vi "Aquisicao_Temperatura_e_Velocidade.vi"() -> ()   [LabVIEW 2018]
uses:
  <vilib>/Analysis/8numeric.llb/1D Numeric Integration.vi
  <vilib>/Waveform/WDTOps.llb/WDT Append Waveforms DBL.vi
  <vilib>/Waveform/WDTOps.llb/WDT Number of Waveform Samples DBL.vi
  <vilib>/Analysis/NI_AALPro.lvlib
panel:
  out "Gráfico de aceleração":waveform(dbl)(graph) caption="Gráfico de temperatura"
  out "Temperatura":dbl format="%#.1g"
  out "stop 2":bool
  in  "Velocidade inicial (m/s)":dbl=1.0 caption="Time Target (s)"
  out "Gráfico de velocidade":waveform(dbl)(graph)
  out "Tempo de aquisição máximo (s) 2":dbl caption="Elapsed Time (s)"
  out "Tempo de aquisição 2 (s)":dbl caption="Elapsed Time (s)"
  in  "Frequência de amostragem (Hz)":dbl=1.0 caption="Time Target (s)"
  out "Tempo de aquisição (s)":dbl caption="Elapsed Time (s)"
  in  "OK Button":bool
  in  "stop":bool
  out "Gráfico de temperatura":waveform(dbl)(graph)
  in  "Unidade de temperatura":enum16{"Celsius", "Kelvin"}(ring)
  in  "Tempo de aquisição máximo (s)":dbl=1.0 caption="Time Target (s)"
  # "CÓDIGO PARA AQUISIÇÃO SINCRONIZADA DE TEMPERATURA E VELOCIDADE"
  # "TEMPERATURA"
  # "VELOCIDADE E ACELERA敲O"
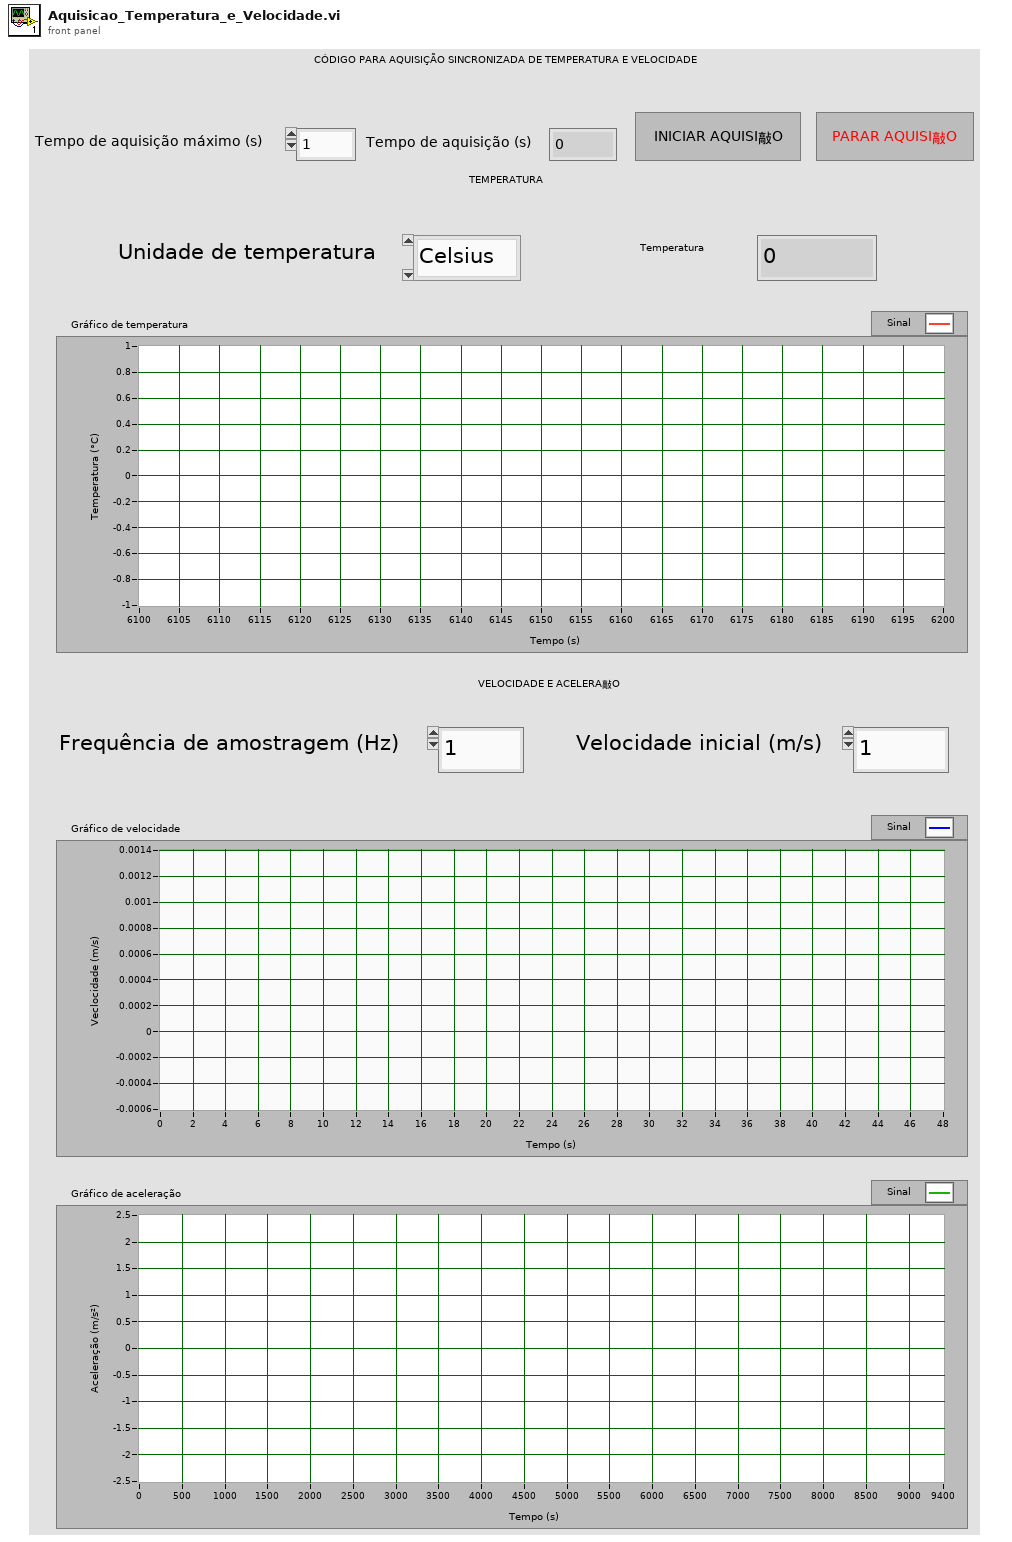
[diagram p1: front panel]
types:
  T1 = typedef "NI_Matrix.lvlib/RealMatrix.ctl" = dbl[][]
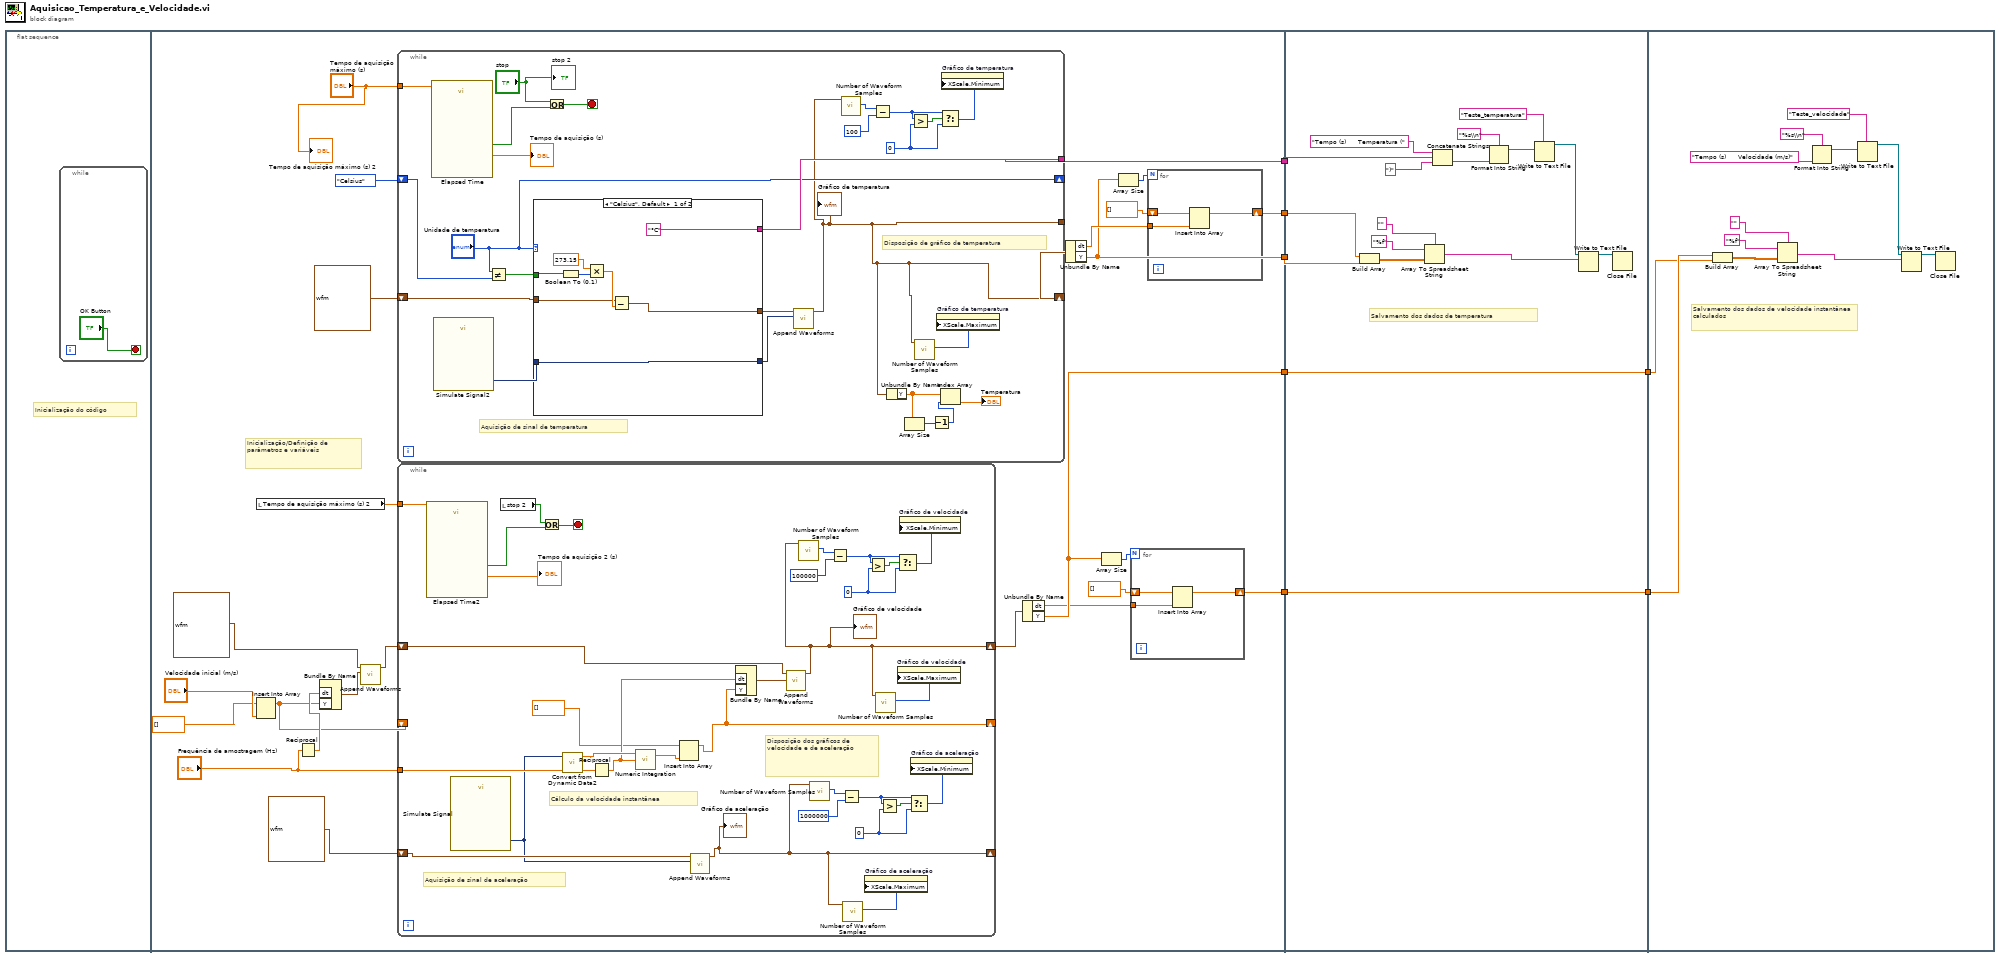
[diagram p0: block diagram]
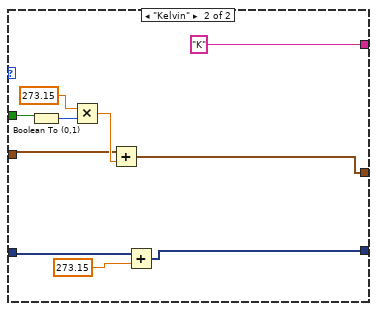
[diagram p2: hidden frame]
diagram:
  n1 = flat-sequence {
    tunnel: [w19] -> w7
    tunnel: [w29] -> w6
    tunnel: [w9] -> w5
    tunnel: [w11] -> w4
    tunnel: [w10] -> w3
    tunnel: w7 -> [w116]
    tunnel: w6 -> [w124]
    tunnel: w5 -> [w118]
    tunnel: w4 -> [w117]
    tunnel: w3 -> [w115]
    tunnel: [w116] -> w2
    tunnel: [w115] -> w1
    tunnel: w2 -> [w132]
    tunnel: w1 -> [w133]
    frame #0 {
      # "Inicialização do código"
      n2 = while {
        stop <- "OK Button" stop-if-true
      }
    }
    frame #1 {
      # "Inicialização/Definição de parâmetros e variáveis"
      n3 = Insert Into Array(array=dbl[] [] ("Y"), new element="Velocidade inicial (m/s)") -> (w23:dbl[])  [unwired: 1 in]
      n4 = local read "Tempo de aquisição máximo (s) 2"() -> (w31:dbl)
      n5 = Reciprocal(x="Frequência de amostragem (Hz)") -> (1/x=w24:dbl)
      n6 = Bundle By Name("dt"=w24, "Y"=w23) -> (w22:waveform(dbl))  [unwired: 1 in]
      n7 = call-poly <vilib>:"Append Waveforms.vi"("waveform B"=w22, "waveform A"=waveform(dbl) {"t0"=timestamp(0 s since 1904-01-01), "dt"=1.0, "Y"=[]}) -> ("waveform out"=w20:waveform(dbl))  [unwired: 8 in, 1 out]
      n8 = while {
        shift-right: [w72] -> w15
        shift-left: waveform(dbl) {"t0"=timestamp(0 s since 1904-01-01), "dt"=1.0, "Y"=[]} ("waveform A") -> [w89]
        tunnel: "Tempo de aquisição máximo (s)" -> [w95]
        shift-right: ["Unidade de temperatura"] -> _
        shift-left: enum16{"Celsius", "Kelvin"}."Celsius" ("Enum") -> [w87]
        tunnel: [w72] -> _
        tunnel: [w93] -> w29
        stop <- w92 stop-if-true
        w75 = 0 ("f")
        # "Disposição de gráfico de temperatura"
        # "Aquisição de sinal de temperatura"
        n9 = call "Elapsed Time"("Time Target (s)"=w95) -> ("Elapsed Time (s)"=→"Tempo de aquisição (s)":dbl, "Time has Elapsed"=w91:bool)  [unwired: 11 in, 6 out]
        n10 = call "Simulate Signal2"() -> ("Sine"=w84:dynamicdata)  [unwired: 14 in, 1 out]
        n11 = Not Equal?(x="Unidade de temperatura", y=w87) -> (x != y?=w86:bool)
        n12 = case shown="\"Celsius\", Default" "Unidade de temperatura" {
          tunnel: ["°C" "K"] -> w93
          tunnel: w89 -> [w99 w105]
          tunnel: [w98 w110] -> w96
          tunnel: w84 -> [w103 w113]
          tunnel: [w103 w112] -> w94
          tunnel: w86 -> [w97 w107]
          frame "Celsius", Default {
            n13 = Boolean To (0,1)(Boolean=w97) -> (0, 1=w101:i16)
            n14 = Multiply(x=273.15 ("y"), y=w101) -> (x*y=w100:dbl)
            n15 = Subtract(x=w99, y=w100) -> (x-y=w98:waveform(dbl))
          }
          frame "Kelvin" {
            n16 = Boolean To (0,1)(Boolean=w107) -> (0, 1=w108:i16)
            n17 = Multiply(x=273.15 ("y"), y=w108) -> (x*y=w106:dbl)
            n18 = Add(x=w105, y=w106) -> (x+y=w110:waveform(dbl))
            n19 = Add(x=w113, y=273.15) -> (x+y=w112:dynamicdata)
          }
        }
        n20 = Or(x="stop", y=w91) -> (x .or. y?=w92:bool)
        n21 = call-poly <vilib>:"Append Waveforms.vi"("waveform B"=w94, "waveform A"=w96) -> ("waveform out"=w72:waveform(dbl))  [unwired: 8 in, 1 out]
        "Gráfico de temperatura" <- w72
        n22 = call-poly <vilib>:"Number of Waveform Samples.vi"("waveform in"=w72) -> ("number of samples"=w79:i32)  [unwired: 8 in, 2 out]
        n23 = Subtract(x=w79, y=100) -> (x-y=w76:i32)
        n24 = Unbundle By Name(w72) -> ("Y"=w83:dbl[])
        n25 = Array Size(array=w83) -> (size(s)=w81:i32)
        n26 = Greater?(x=w76, y=w75) -> (0:w77:bool)
        n27 = call-poly <vilib>:"Number of Waveform Samples.vi"("waveform in"=w72) -> ("number of samples"=w73:i32)  [unwired: 8 in, 2 out]
        n28 = Decrement(x=w81) -> (x-1=w80:i32)
        n29 = property on="Gráfico de temperatura" class="WFGraph (strict)"("XScale.Maximum"=w73) -> ()  [unwired: 2 in, 2 out]
        n30 = Select(t=w76, s=w77, f=w75) -> (s? t:f=w74:i32)
        n31 = Index Array(array=w83, index=w80) -> (element=→"Temperatura":dbl)
        n32 = property on="Gráfico de temperatura" class="WFGraph (strict)"("XScale.Minimum"=w74) -> ()  [unwired: 2 in, 2 out]
        "stop 2" <- "stop"
      }
      n33 = while {
        tunnel: w31 -> [w70]
        tunnel: "Frequência de amostragem (Hz)" -> [w42]
        shift-right: [w51] -> w30
        shift-left: w20 -> [w52]
        shift-right: [w43] -> _
        shift-left: waveform(dbl) {"t0"=timestamp(0 s since 1904-01-01), "dt"=1.0, "Y"=[]} ("waveform A") -> [w66]
        shift-right: [w54] -> _
        shift-left: w23 -> [_]
        stop <- w69 stop-if-true
        w46 = 0 ("f")
        w61 = 0 ("f")
        # "Disposição dos gráficos de velocidade e de aceleração"
        # "Cálculo da velocidade instantânea"
        # "Aquisição de sinal de aceleração"
        n34 = call "Elapsed Time2"("Time Target (s)"=w70) -> ("Elapsed Time (s)"=→"Tempo de aquisição 2 (s)":dbl, "Time has Elapsed"=w71:bool)  [unwired: 11 in, 6 out]
        n35 = call "Simulate Signal"() -> ("Sine with Uniform Noise"=w41:dynamicdata)  [unwired: 14 in, 1 out]
        n36 = local read "stop 2"() -> (w67:bool)
        n37 = Or(x=w67, y=w71) -> (x .or. y?=w69:bool)
        n38 = call "Convert from Dynamic Data2"("Dynamic Data Type"=w41) -> ("Array"=w58:dbl[])  [unwired: 3 in]
        n39 = Reciprocal(x=w42) -> (1/x=w57:dbl)
        n40 = call-poly <vilib>:"Numeric Integration.vi"("dt"=w57, "Input Array"=w58) -> ("result"=w56:dbl)  [unwired: 1 in, 1 out]
        n41 = Insert Into Array(array=dbl[] [] ("Y"), new element=w56) -> (w54:dbl[])  [unwired: 1 in]
        n42 = call-poly <vilib>:"Append Waveforms.vi"("waveform B"=w41, "waveform A"=w66) -> ("waveform out"=w43:waveform(dbl))  [unwired: 8 in, 1 out]
        "Gráfico de aceleração" <- w43
        n43 = Bundle By Name("dt"=w57, "Y"=w54) -> (w53:waveform(dbl))  [unwired: 1 in]
        n44 = call-poly <vilib>:"Append Waveforms.vi"("waveform B"=w53, "waveform A"=w52) -> ("waveform out"=w51:waveform(dbl))  [unwired: 8 in, 1 out]
        "Gráfico de velocidade" <- w51
        n45 = call-poly <vilib>:"Number of Waveform Samples.vi"("waveform in"=w51) -> ("number of samples"=w65:i32)  [unwired: 8 in, 2 out]
        n46 = call-poly <vilib>:"Number of Waveform Samples.vi"("waveform in"=w43) -> ("number of samples"=w50:i32)  [unwired: 8 in, 2 out]
        n47 = Subtract(x=w65, y=100000) -> (x-y=w62:i32)
        n48 = Subtract(x=w50, y=1000000) -> (x-y=w47:i32)
        n49 = call-poly <vilib>:"Number of Waveform Samples.vi"("waveform in"=w43) -> ("number of samples"=w44:i32)  [unwired: 8 in, 2 out]
        n50 = property on="Gráfico de aceleração" class="WFGraph (strict)"("XScale.Maximum"=w44) -> ()  [unwired: 2 in, 2 out]
        n51 = Greater?(x=w62, y=w61) -> (0:w63:bool)
        n52 = call-poly <vilib>:"Number of Waveform Samples.vi"("waveform in"=w51) -> ("number of samples"=w59:i32)  [unwired: 8 in, 2 out]
        n53 = Greater?(x=w47, y=w46) -> (0:w48:bool)
        n54 = property on="Gráfico de velocidade" class="WFGraph (strict)"("XScale.Maximum"=w59) -> ()  [unwired: 2 in, 2 out]
        n55 = Select(t=w62, s=w63, f=w61) -> (s? t:f=w60:i32)
        n56 = property on="Gráfico de velocidade" class="WFGraph (strict)"("XScale.Minimum"=w60) -> ()  [unwired: 2 in, 2 out]
        n57 = Select(t=w47, s=w48, f=w46) -> (s? t:f=w45:i32)
        n58 = property on="Gráfico de aceleração" class="WFGraph (strict)"("XScale.Minimum"=w45) -> ()  [unwired: 2 in, 2 out]
      }
      n59 = Unbundle By Name(w30) -> ("dt"=w17:dbl, "Y"=w19:dbl[])
      n60 = Unbundle By Name(w15) -> ("dt"=w12:dbl, "Y"=w9:dbl[])
      n61 = Array Size(array=w19) -> (size(s)=w16:i32)
      n62 = Array Size(array=w9) -> (size(s)=w13:i32)
      n63 = for {
        N: w16 -> [_]
        shift-right: [w39] -> w10
        shift-left: dbl[] [] ("array") -> [w40]
        tunnel: w17 -> [w38]
        n64 = Insert Into Array(array=w40, new element=w38) -> (w39:dbl[])  [unwired: 1 in]
      }
      n65 = for {
        N: w13 -> [_]
        shift-right: [w36] -> w11
        shift-left: dbl[] [] ("array") -> [w37]
        tunnel: w12 -> [w35]
        n66 = Insert Into Array(array=w37, new element=w35) -> (w36:dbl[])  [unwired: 1 in]
      }
      "Tempo de aquisição máximo (s) 2" <- "Tempo de aquisição máximo (s)"
    }
    frame #2 {
      # "Salvamento dos dados de temperatura"
      n67 = Build Array(w117, w118) -> (w120:T1)
      n68 = Array To Spreadsheet String(delimiter (Tab)="", array=w120, 3:"%f" ("format string")) -> (spreadsheet string=w119:string)
      n69 = Concatenate Strings("Tempo (s)      Temperatura (" ("string"), w124, ")" ("string")) -> (w128:string)
      n70 = Format Into String(format string="%s\\n" ("initial string"), w128) -> (resulting string=w129:string)  [unwired: 2 in, 1 out]
      n71 = Write to Text File(prompt (Choose or enter file path)="Teste_temperatura", text=w129) -> (refnum out=w130:refnum<file>)  [unwired: 2 in, 2 out]
      n72 = Write to Text File(file (use dialog)=w130, text=w119) -> (refnum out=w131:refnum<file>)  [unwired: 2 in, 2 out]
      n73 = Close File(refnum=w131) -> ()  [unwired: 1 in, 2 out]
    }
    frame #3 {
      # "Salvamento dos dados de velocidade instantânea calculados"
      n74 = Build Array(w133, w132) -> (w137:T1)
      n75 = Array To Spreadsheet String(delimiter (Tab)="", array=w137, 3:"%f" ("format string")) -> (spreadsheet string=w136:string)
      n76 = Format Into String(format string="%s\\n" ("initial string"), "Tempo (s)      Velocidade (m/s)" ("string")) -> (resulting string=w141:string)  [unwired: 2 in, 1 out]
      n77 = Write to Text File(prompt (Choose or enter file path)="Teste_velocidade", text=w141) -> (refnum out=w142:refnum<file>)  [unwired: 2 in, 2 out]
      n78 = Write to Text File(file (use dialog)=w142, text=w136) -> (refnum out=w143:refnum<file>)  [unwired: 2 in, 2 out]
      n79 = Close File(refnum=w143) -> ()  [unwired: 1 in, 2 out]
    }
  }
